vi "Meta.vi"(7 "LabVIEW Web Service Request":refnum<class "Web Request.lvclass">, 11 "expId":string) -> ()   [LabVIEW 2015]
uses:
  <vilib>/wsapi/Web Request.lvclass
  Configuration/Global_Configurations.vi
panel:
  # "Use the Web Service Request input terminal to call the VIs on the Web Services palette. Do not remove it from the connector pane unless you don't need access to the palette."
  # "Each additional control wired to the connector pane will be available as an input in the URL. To include an indicator in terminal-mode output (the default setting), it must also be wired to the connector pane."
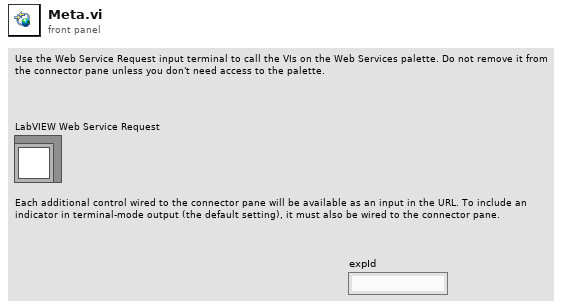
[diagram p1: front panel]
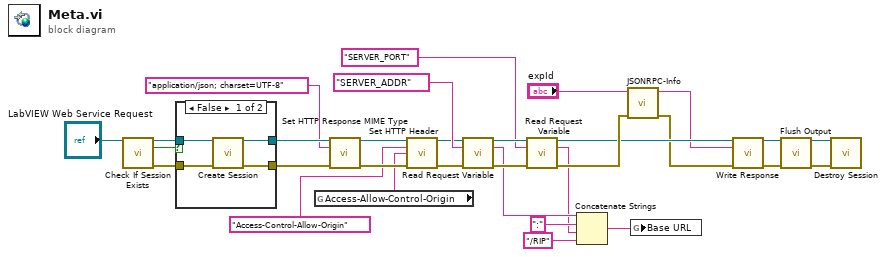
[diagram p0: block diagram]
diagram:
  n1 = call <vilib>:"Check If Session Exists.vi"("LabVIEW Web Service Request"="LabVIEW Web Service Request") -> ("LabVIEW Web Service Request out"=w31:refnum<class "Web Request.lvclass">, "session exists?"=w30:bool, "error out"=w29:errorcluster)  [unwired: 12 in]
  n2 = case shown="False" w30 {
    tunnel: w31 -> [w35 w37]
    tunnel: [w34 w37] -> w12
    tunnel: w29 -> [w33 w36]
    tunnel: [w32 w36] -> w11
    frame False {
      n3 = call <vilib>:"Create Session.vi"("LabVIEW Web Service Request"=w35, "error in (no error)"=w33) -> ("LabVIEW Web Service Request out"=w34:refnum<class "Web Request.lvclass">, "error out"=w32:errorcluster)  [unwired: 11 in, 1 out]
    }
    frame True {
    }
  }
  n4 = global read "Global_Configurations.vi" "Access-Allow-Control-Origin"() -> (w1:string)
  n5 = call <vilib>:"Set HTTP Response MIME Type.vi"("LabVIEW Web Service Request"=w12, "MIME type (text/html)"="application/json; charset=UTF-8" ("header"), "error in (no error)"=w11) -> ("LabVIEW Web Service Request out"=w14:refnum<class "Web Request.lvclass">, "error out"=w13:errorcluster)  [unwired: 11 in]
  n6 = call <vilib>:"Set HTTP Header.vi"("LabVIEW Web Service Request"=w14, "header"="Access-Control-Allow-Origin", "header value"=w1, "error in (no error)"=w13) -> ("LabVIEW Web Service Request out"=w10:refnum<class "Web Request.lvclass">, "error out"=w9:errorcluster)  [unwired: 10 in]
  n7 = call <vilib>:"Read Request Variable.vi"("LabVIEW Web Service Request"=w10, "variable name"="SERVER_ADDR", "error in (no error)"=w9) -> ("LabVIEW Web Service Request out"=w22:refnum<class "Web Request.lvclass">, "value"=w17:string, "error out"=w21:errorcluster)  [unwired: 10 in]
  n8 = call <vilib>:"Read Request Variable.vi"("LabVIEW Web Service Request"=w22, "variable name"="SERVER_PORT", "error in (no error)"=w21) -> ("LabVIEW Web Service Request out"=w7:refnum<class "Web Request.lvclass">, "value"=w16:string, "error out"=w19:errorcluster)  [unwired: 10 in]
  n9 = Concatenate Strings(w17, ":" ("string"), w16, "/RIP" ("string")) -> (w3:string)
  n10 = call "JSONRPC-Info.vi"("error in (no error)"=w19, "info"="expId") -> ("error out"=w4:errorcluster, "result"=w5:string)  [unwired: 8 in]
  n11 = global write "Global_Configurations.vi" "Base URL"(w3) -> ()
  n12 = call <vilib>:"Write Response.vi"("LabVIEW Web Service Request"=w7, "response string"=w5, "error in (no error)"=w4) -> ("LabVIEW Web Service Request out"=w26:refnum<class "Web Request.lvclass">, "error out"=w27:errorcluster)  [unwired: 11 in]
  n13 = call <vilib>:"Flush Output.vi"("LabVIEW Web Service Request"=w26, "error in (no error)"=w27) -> ("LabVIEW Web Service Request out"=w25:refnum<class "Web Request.lvclass">, "error out"=w24:errorcluster)  [unwired: 12 in]
  n14 = call <vilib>:"Destroy Session.vi"("LabVIEW Web Service Request"=w25, "error in (no error)"=w24) -> ()  [unwired: 12 in, 2 out]
